vi "sendMessage.vi"(8 "error in (no error)":errorcluster, 10 "Message":string, 11 "User in":refnum<class "User.lvclass">) -> (0 "error out":errorcluster, 3 "User out":refnum<class "User.lvclass">)   [LabVIEW 2016, in "User.lvclass"]
uses:
  User.lvclass
  ChatRoom/ChatRoom.lvclass
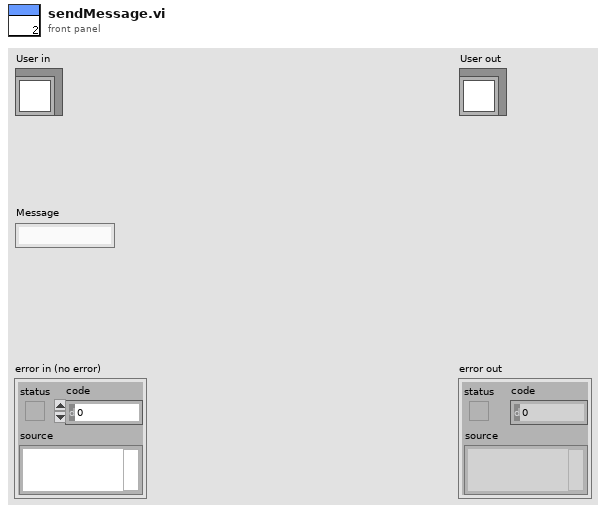
[diagram p1: front panel]
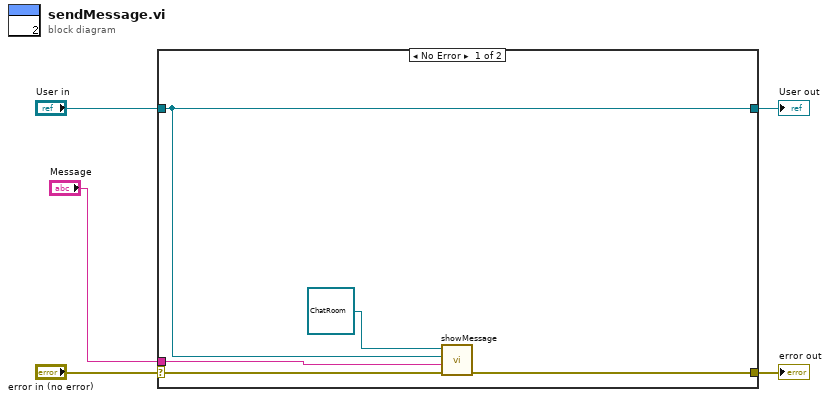
[diagram p0: block diagram]
diagram:
  n1 = case shown="No Error" "error in (no error)" {
    selector: "error in (no error)" -> [w10 w12]
    tunnel: [w9 w12] -> w4
    tunnel: [w6 w11] -> w2
    tunnel: "User in" -> [w6 w11]
    tunnel: "Message" -> [w7 _]
    frame No Error {
      n2 = call "showMessage.vi"("error in (no error)"=w10, "Message"=w7, "User.lvclass"=w6, "ChatRoom in"=refnum<class "ChatRoom.lvclass"> refnum ("ChatRoom.lvclass")) -> ("error out"=w9:errorcluster)  [unwired: 6 in, 1 out]
    }
    frame Error {
    }
  }
  "error out" <- w4
  "User out" <- w2
